vi "TestButtonPulse.vi"() -> ()   [LabVIEW 2017]
panel:
  in  "Number of milliseconds to wait.\n~20ms precision.":i32=12
  in  "Input":bool
  out "RisingPulse":bool
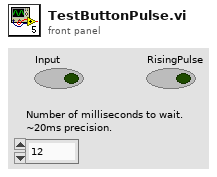
[diagram p1: front panel]
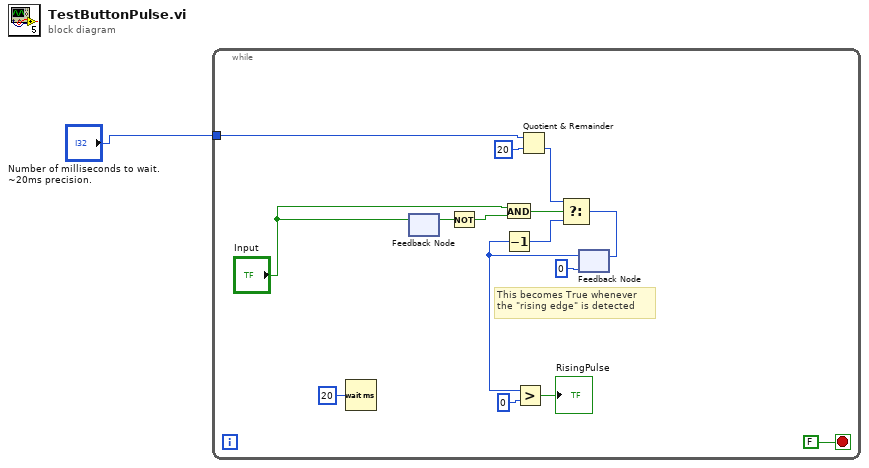
[diagram p0: block diagram]
diagram:
  n1 = while {
    tunnel: "Number of milliseconds to wait.\n~20ms precision." -> [w5]
    stop <- FALSE stop-if-true
    # "This becomes True whenever \nthe \"rising edge\" is detected"
    n2 = Wait (ms)(milliseconds to wait=u32 20) -> ()  [unwired: 1 out]
    n3 = feedback #1() -> (w10:bool)  [unwired: 1 in]
    n4 = feedback-in #1("Input") -> ()
    n5 = Not(x=w10) -> (.not. x?=w11:bool)
    n6 = And(x="Input", y=w11) -> (x .and. y?=w9:bool)
    n7 = Quotient & Remainder(x=w5, y=20) -> (floor(x/y)=w12:i32)  [unwired: 1 out]
    n8 = feedback #2(0 ("Number of loops to wait \nbetween each change.")) -> (w8:i32)
    n9 = Decrement(x=w8) -> (x-1=w14:i32)
    n10 = Greater?(x=w8, y=0 ("x")) -> (0:→"RisingPulse":bool)
    n11 = Select(t=w12, s=w9, f=w14) -> (s? t:f=w15:i32)
    n12 = feedback-in #2(w15) -> ()
  }
